vi "Authorize.vi"(6 "timeout (ms) [0: default]":i32, 8 "error in (no error)":errorcluster, 10 "State Parameter":string, 11 "Oauth2 in":refnum<class "Oauth2.lvclass">) -> (0 "error out":errorcluster, 2 "Access Token":string, 3 "Oauth2 out":refnum<class "Oauth2.lvclass">)   [LabVIEW 2017, in "Oauth2.lvclass"]
uses:
  Oauth2.lvclass
  OAuthToken/OAuth2 Token Element -- enum.ctl
  Oauth2.lvclass/Oauth2.ctl
  OAuth2 Grant Type -- ring.ctl
  <vilib>/LabVIEW Open Source Project/OpenURI/uri/URI.lvclass/URI.ctl
  OauthClient/OAuthClient.lvclass/OAuthClient.ctl
  <vilib>/LabVIEW Open Source Project/Connection/Connection.TCP/Connection.TCP.lvclass
  C:/Program Files (x86)/National Instruments/LabVIEW 2024/vi.lib/LabVIEW Open Source Project/Connection/Connection/Connection.lvclass
  <vilib>/LabVIEW Open Source Project/Connection/Connection/Connection.lvclass
  <vilib>/LabVIEW Open Source Project/OpenURI/uri/URI.lvclass
  OAuthToken/OAuthAccessToken.lvclass
  OauthClient/OAuthClient.lvclass
panel:
  in  "Status":string(combo)="400 BAD REQUEST"
  out "Request":string
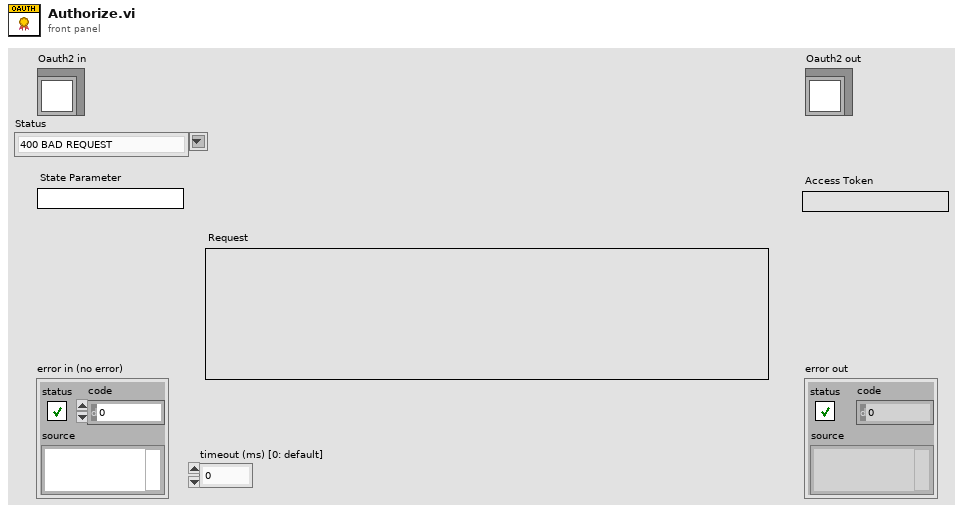
[diagram p1: front panel]
types:
  T1 = typedef "OAuthAccessToken.lvclass/OAuth2 Token Element -- enum.ctl" = enum16{"client_id", "client_secret", "response_type", "scope", "redirect_uri", "error", "error_description", "error_uri", "grant_type", "code", "access_token", "token_type", "expires_in", "username", "password", "refresh_token", "code_challenge", "code_challenge_method", "reverse_proxy_uri", "endpoint element", "access_type", "prompt", "id_token"}
  T2 = typedef "Oauth2.lvclass/OAuth2 Flow -- enum.ctl" = enum16{"Authorization Code", "Authorization Code (PKCE)", "Implicit", "Resource Owner Credentials", "Client Credentials"}
  T3 = typedef "Oauth2.lvclass/OAuth2 Grant Type -- ring.ctl" = string
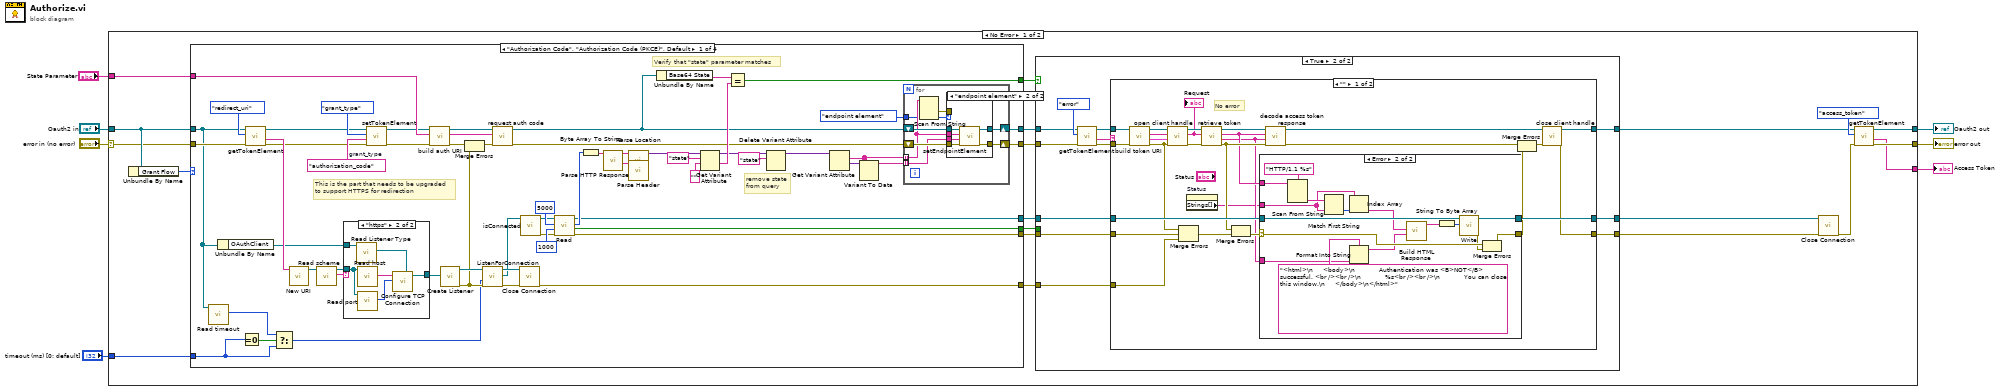
[diagram p0: block diagram]
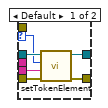
[diagram p2: hidden frame]
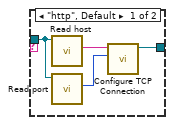
[diagram p3: hidden frame]
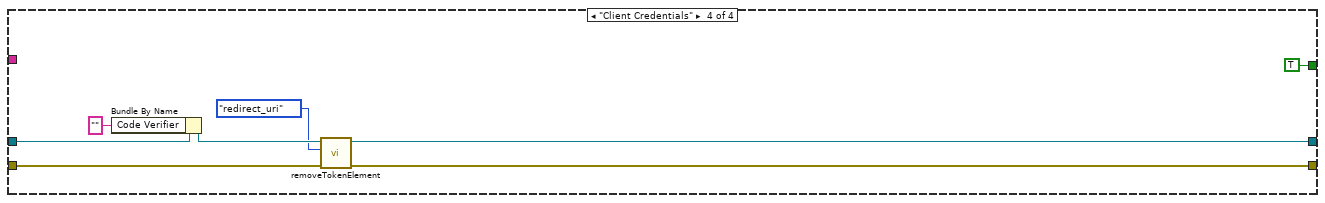
[diagram p6: hidden frame]
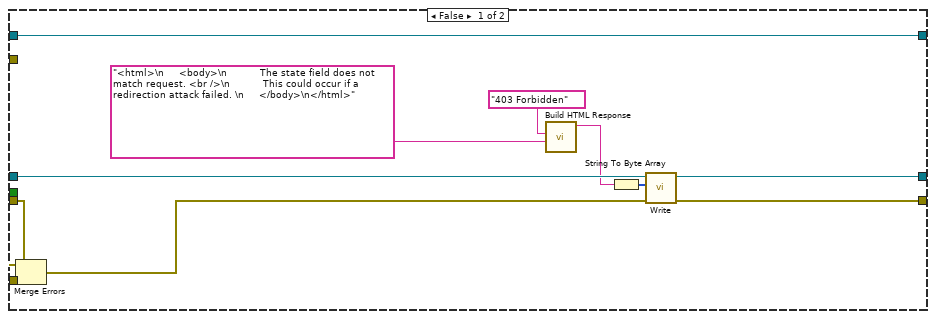
[diagram p7: hidden frame]
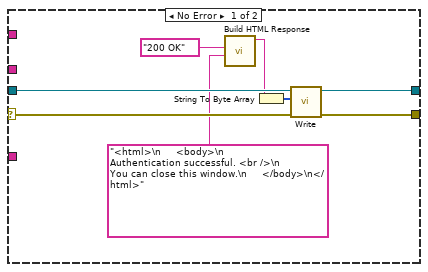
[diagram p8: hidden frame]
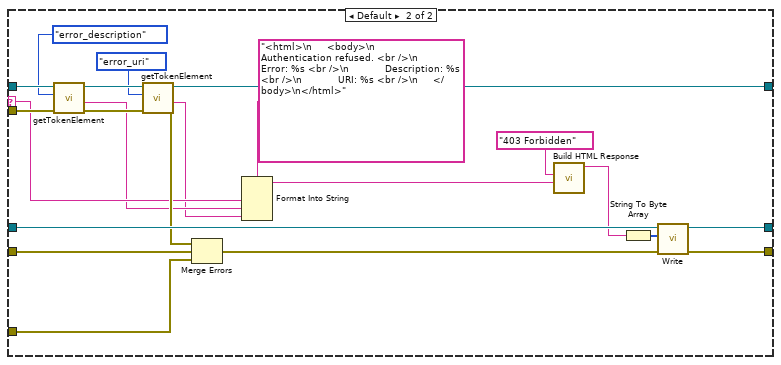
[diagram p9: hidden frame]
diagram:
  n1 = case shown="No Error" "error in (no error)" {
    selector: "error in (no error)" -> [w8 w226]
    tunnel: [w17 w226] -> w6
    tunnel: [w19 w225] -> w4
    tunnel: "Oauth2 in" -> [w9 w225]
    tunnel: "State Parameter" -> [w27 _]
    tunnel: [w14 _] -> w2
    tunnel: "timeout (ms) [0: default]" -> [w13 _]
    frame No Error {
      n2 = Unbundle By Name(w9) -> ("Grant Flow"=w10:T2)
      n3 = case shown="\"Authorization Code\", \"Authorization Code (PKCE)\", Default" w10 {
        tunnel: w27 -> [w83 _ _ _]
        tunnel: [w67 _ _ _] -> w25
        tunnel: [w66 _ _ _] -> w24
        tunnel: [w65 _ _ _] -> w23
        tunnel: [w61 _ _ TRUE] -> w21
        tunnel: [w60 _ _ _] -> w20
        tunnel: w13 -> [w43 _ _ _]
        tunnel: [w31 w118 w120 w122] -> w12
        tunnel: [w30 w117 w119 w121] -> w11
        tunnel: w8 -> [w29 w117 w119 w123]
        tunnel: w9 -> [w28 w118 w120 w127]
        frame "Authorization Code", "Authorization Code (PKCE)", Default {
          w46 = T3 "authorization_code"  # grant_type
          # "This is the part that needs to be upgraded\nto support HTTPS for redirection"
          # "remove state\nfrom query"
          # "Verify that \"state\" parameter matches"
          n4 = call "Read timeout.vi"("Oauth2 in"=w28) -> ("timeout (ms)"=w41:i32)  [unwired: 8 in, 2 out]
          n5 = Unbundle By Name(w28) -> ("OAuthClient"=w39:refnum<class "OAuthClient.lvclass">)
          n6 = Equal To 0?(x=w43) -> (x = 0?=w64:bool)
          n7 = call "getTokenElement.vi"("error in (no error)"=w29, "Token element"=OAuth2_Token_Element_--_enum."redirect_uri", "Oauth2 in"=w28) -> ("error out"=w42:errorcluster, "Value"=w58:string, "Oauth2 out"=w40:refnum<class "Oauth2.lvclass">)  [unwired: 4 in, 2 out]
          n8 = Select(t=w41, s=w64, f=w43) -> (s? t:f=w63:i32)
          n9 = call <vilib>:"New URI.vi"("URI"=w58) -> ("URI"=w57:refnum<class "URI.lvclass">)  [unwired: 9 in, 1 out]
          n10 = call <vilib>:"Read scheme.vi"("URI in"=w57) -> ("scheme"=w85:string, "URI out"=w84:refnum<class "URI.lvclass">)  [unwired: 8 in, 1 out]
          n11 = case shown="\"https\"" w85 {
            tunnel: w84 -> [w107 w113]
            tunnel: [w108 w114] -> w74
            tunnel: w39 -> [_ w112]
            frame "http", Default {
              n12 = call <vilib>:"Read host.vi"("URI in"=w107) -> ("host"=w110:string)  [unwired: 8 in, 2 out]
              n13 = call <vilib>:"Read port.vi"("URI in"=w107) -> ("port"=w109:u16)  [unwired: 8 in, 2 out]
              n14 = call <vilib>:"Configure TCP Connection.vi"("remote port (80)"=w109, "address (localhost)"=w110) -> ("Connection.TCP"=w108:refnum<class "Connection.TCP.lvclass">)  [unwired: 8 in, 1 out]
            }
            frame "https" {
              n15 = call "Read Listener Type.vi"("OAuthClient in"=w112) -> ("Listener Type"=w111:refnum<class "Connection.TCP.lvclass">)  [unwired: 8 in, 2 out]
              n16 = call <vilib>:"Read host.vi"("URI in"=w113) -> ("host"=w116:string)  [unwired: 8 in, 2 out]
              n17 = call <vilib>:"Read port.vi"("URI in"=w113) -> ("port"=w115:u16)  [unwired: 8 in, 2 out]
              n18 = call <vilib>:"Configure TCP Connection.vi"("Connection.TCP"=w111, "remote port (80)"=w115, "address (localhost)"=w116) -> ("Connection.TCP"=w114:refnum<class "Connection.TCP.lvclass">)  [unwired: 7 in, 1 out]
            }
          }
          n19 = call "setTokenElement.vi"("error in (no error)"=w42, "Value"=w46, "Token element"=OAuth2_Token_Element_--_enum."grant_type", "Oauth2 in"=w40) -> ("error out"=w44:errorcluster, "Oauth2 out"=w45:refnum<class "Oauth2.lvclass">)  [unwired: 6 in]
          n20 = call-dynamic "build auth URI.vi"("error in (no error)"=w44, "State Parameter"=w83, "Oauth2 in"=w45) -> ("error out"=w68:errorcluster, "Authorization Request URI"=w70:string, "Oauth2"=w69:refnum<class "Oauth2.lvclass">)  [unwired: 6 in]
          n21 = call <vilib>:"Create Listener.vi"("Connection Configuration"=w74) -> ("error out"=w72:errorcluster, "Listener"=w80:refnum<class "Connection.TCP.lvclass">)  [unwired: 9 in]
          n22 = Merge Errors(w68, w72) -> (w71:errorcluster)
          n23 = call <vilib>:"ListenForConnection.vi"("error in (no error)"=w72, "timeout (2000 ms)"=w63, "Listener"=w80) -> ("error out"=w82:errorcluster, "Connection"=w77:refnum<class "Connection.lvclass">, "Listener out"=w79:refnum<class "Connection.TCP.lvclass">)  [unwired: 5 in, 1 out]
          n24 = call-dynamic "request auth code.vi"("error in (no error)"=w71, "Request URI"=w70, "Oauth2 in"=w69) -> ("error out"=w33:errorcluster, "Oauth2 out"=w34:refnum<class "Oauth2.lvclass">)  [unwired: 7 in]
          n25 = call <vilib>:"Close Connection.vi"("error in (no error)"=w82, "Connection in"=w79) -> ("error out"=w66:errorcluster)  [unwired: 8 in, 1 out]
          n26 = call <vilib>:"isConnected.vi"("Connection in"=w77) -> ("error out"=w75:errorcluster, "Connection out"=w76:refnum<class "Connection.lvclass">)  [unwired: 8 in, 1 out]
          n27 = call <vilib>:"Read.vi"("error in (no error)"=w75, "timeout (2000 ms)"=1000 ("bytes to read (100)"), "bytes to read (100)"=5000, "TCPConnection in"=w76) -> ("error out"=w65:errorcluster, "timed out"=w60:bool, "Bytes"=w73:u8[], "TCPConnection out"=w67:refnum<class "Connection.lvclass">)  [unwired: 3 in, 1 out]
          n28 = Byte Array To String(unsigned byte array=w73) -> (string=w56:string)
          n29 = call "Parse HTTP Response.vi"("HTTP Response"=w56) -> ("Header"=w55:string, "Location"=w54:string)  [unwired: 5 in, 4 out]
          n30 = call "Parse Location.vi"("Location"=w54) -> ("Query Parameters"=w53:variant)  [unwired: 10 in]
          n31 = call "Parse Header.vi"("HTTP Header"=w55) -> ()  [unwired: 10 in, 1 out]
          n32 = Unbundle By Name(w34) -> ("Base64 State"=w62:string)
          n33 = Get Variant Attribute(Variant=w53, name="state", default value (empty Variant)="") -> (duplicate Variant=w49:variant, value=w50:string)  [unwired: 1 in, 2 out]
          n34 = Equal?(x=w62, y=w50) -> (x = y?=w61:bool)
          n35 = Delete Variant Attribute(6:"state", 7:w49) -> (3:w32:variant)  [unwired: 1 in, 2 out]
          n36 = Get Variant Attribute(Variant=w32) -> (names=w38:string[], values=w36:variant[])  [unwired: 3 in, 2 out]
          n37 = Variant To Data(type=w38, Variant=w36) -> (data=w37:string[])  [unwired: 1 in, 1 out]
          n38 = for {
            shift-right: [w92] -> w31
            shift-left: w34 -> [w93]
            shift-right: [w89] -> w30
            shift-left: w33 -> [w91]
            tunnel: w38 -> [w87] mode=indexing
            tunnel: w37 -> [w90] mode=indexing
            tunnel: OAuth2_Token_Element_--_enum."endpoint element" ("Token element") -> [w86]
            n39 = Scan From String(input string=w87, default 1=w86) -> (error out=w88:errorcluster, output 1=w94:T1)  [unwired: 3 in, 2 out]
            n40 = case shown="\"endpoint element\"" w94 {
              selector: w94 -> [w98 _]
              tunnel: w93 -> [w100 w106]
              tunnel: [w99 w105] -> w92
              tunnel: w91 -> [w97 w104]
              tunnel: w90 -> [w96 w102]
              tunnel: [w95 w103] -> w89
              tunnel: w88 -> [_ _]
              tunnel: w87 -> [_ w101]
              frame Default {
                n41 = call "setTokenElement.vi"("error in (no error)"=w97, "Value"=w96, "Token element"=w98, "Oauth2 in"=w100) -> ("error out"=w95:errorcluster, "Oauth2 out"=w99:refnum<class "Oauth2.lvclass">)  [unwired: 6 in]
              }
              frame "endpoint element" {
                n42 = call "setEndpointElement.vi"("error in (no error)"=w104, "Value"=w102, "Endpoint Name"=w101, "Oauth2 in"=w106) -> ("error out"=w103:errorcluster, "Oauth2 out"=w105:refnum<class "Oauth2.lvclass">)  [unwired: 6 in]
              }
            }
          }
        }
        frame "Implicit" {
        }
        frame "Resource Owner Credentials" {
        }
        frame "Client Credentials" {
          n43 = Bundle By Name(cluster=w127, "Code Verifier"="") -> (w126:refnum<class "Oauth2.lvclass">)
          n44 = call "removeTokenElement.vi"("error in (no error)"=w123, "Token element"=OAuth2_Token_Element_--_enum."redirect_uri", "Oauth2 in"=w126) -> ("error out"=w121:errorcluster, "Oauth2 out"=w122:refnum<class "Oauth2.lvclass">)  [unwired: 7 in]
        }
      }
      n45 = case shown="True" w21 {
        tunnel: w12 -> [w133 w142]
        tunnel: w11 -> [w132 w141]
        tunnel: [w138 w152] -> w26
        tunnel: w25 -> [w139 w151]
        tunnel: w24 -> [w136 w150]
        tunnel: w23 -> [w135 w149]
        tunnel: [w133 w148] -> w15
        tunnel: [w137 w147] -> w22
        tunnel: w20 -> [_ _]
        frame False {
          n46 = Merge Errors(w132, w135, w136) -> (w134:errorcluster)
          n47 = call "Build HTML Response.vi"("HTML"="<html>\n     <body>\n           The state field does not match request. <br />\n           This could occur if a redirection attack failed. \n     </body>\n</html>" ("regular expression"), "Status"="403 Forbidden") -> ("HTTP Response"=w129:string)  [unwired: 9 in]
          n48 = String To Byte Array(string=w129) -> (unsigned byte array=w140:u8[])
          n49 = call <vilib>:"Write.vi"("error in (no error)"=w134, "Bytes"=w140, "Connection in"=w139) -> ("error out"=w137:errorcluster, "Connection"=w138:refnum<class "Connection.lvclass">)  [unwired: 7 in]
        }
        frame True {
          n50 = call "getTokenElement.vi"("error in (no error)"=w141, "Token element"=OAuth2_Token_Element_--_enum."error", "Oauth2 in"=w142) -> ("error out"=w145:errorcluster, "Value"=w143:string, "Oauth2 out"=w146:refnum<class "Oauth2.lvclass">)  [unwired: 4 in, 2 out]
          n51 = case shown="\"\"" w143 {
            selector: w143 -> [_ w209]
            tunnel: [w178 w224] -> w152
            tunnel: w151 -> [w177 w222]
            tunnel: w150 -> [w176 w221]
            tunnel: w149 -> [w175 w220]
            tunnel: [w169 w214] -> w148
            tunnel: [w161 w219] -> w147
            tunnel: w146 -> [w160 w217]
            tunnel: w145 -> [w159 w212]
            frame "" {
              # "No error"
              n52 = call-dynamic "build token URI.vi"("error in (no error)"=w159, "Oauth2 in"=w160) -> ("error out"=w171:errorcluster, "Headers"=w158:cluster{"header":string, "value":string}[], "Token Request URI"=w172:string, "Oauth2"=w173:refnum<class "Oauth2.lvclass">)  [unwired: 6 in]
              n53 = call "open client handle.vi"("error in (no error)"=w171, "Headers"=w158, "Request URI in"=w172, "Oauth2 in"=w173) -> ("error out"=w167:errorcluster, "Request URI dup"=w166:string, "Oauth2 out"=w168:refnum<class "Oauth2.lvclass">)  [unwired: 5 in]
              "Request" <- w166
              n54 = Merge Errors(w171, w175, w176) -> (w174:errorcluster)
              n55 = property on="Status" class="CmbBox"() -> ("Strings[]"=w153:string[])  [unwired: 2 in, 2 out]
              n56 = call "retrieve token.vi"("error in (no error)"=w167, "Token Request URI"=w166, "Oauth2 in"=w168) -> ("error out"=w163:errorcluster, "Response"=w154:string, "Header"=w155:string, "Oauth2 out"=w165:refnum<class "Oauth2.lvclass">)  [unwired: 5 in]
              n57 = Merge Errors(w163, w174) -> (w156:errorcluster)
              n58 = case shown="Error" w156 {
                selector: w156 -> [w182 w199]
                tunnel: [w186 w202] -> w178
                tunnel: w177 -> [w184 w200]
                tunnel: [w183 w197] -> w157
                tunnel: w155 -> [_ w195]
                tunnel: w154 -> [_ w188]
                tunnel: w153 -> [_ w190]
                frame No Error {
                  n59 = call "Build HTML Response.vi"("HTML"="<html>\n     <body>\n            Authentication successful. <br />\n            You can close this window.\n     </body>\n</html>" ("regular expression"), "Status"="200 OK") -> ("HTTP Response"=w180:string)  [unwired: 9 in]
                  n60 = String To Byte Array(string=w180) -> (unsigned byte array=w185:u8[])
                  n61 = call <vilib>:"Write.vi"("error in (no error)"=w182, "Bytes"=w185, "Connection in"=w184) -> ("error out"=w183:errorcluster, "Connection"=w186:refnum<class "Connection.lvclass">)  [unwired: 7 in]
                }
                frame Error {
                  n62 = Scan From String(format string="HTTP/1.1 %s", input string=w195) -> (output 1=w193:string)  [unwired: 3 in, 3 out]
                  n63 = Match First String(2:w190, 3:w193) -> (0:w192:i32)  [unwired: 1 out]
                  n64 = Index Array(array=w190, index=w192) -> (element=w191:string)
                  n65 = Format Into String(format string="<html>\n     <body>\n            Authentication was <B>NOT</B> successful. <br /><br />\n            %s<br /><br />\n            You can close this window.\n     </body>\n</html>" ("regular expression"), w188) -> (resulting string=w187:string)  [unwired: 2 in, 1 out]
                  n66 = call "Build HTML Response.vi"("HTML"=w187, "Status"=w191) -> ("HTTP Response"=w196:string)  [unwired: 9 in]
                  n67 = String To Byte Array(string=w196) -> (unsigned byte array=w201:u8[])
                  n68 = call <vilib>:"Write.vi"("Bytes"=w201, "Connection in"=w200) -> ("error out"=w198:errorcluster, "Connection"=w202:refnum<class "Connection.lvclass">)  [unwired: 8 in]
                  n69 = Merge Errors(w199, w198) -> (w197:errorcluster)
                }
              }
              n70 = call-dynamic "decode access token response.vi"("error in (no error)"=w163, "Response"=w154, "Header"=w155, "Oauth2 in"=w165) -> ("error out"=w162:errorcluster, "Oauth2"=w164:refnum<class "Oauth2.lvclass">)  [unwired: 6 in]
              n71 = Merge Errors(w162, w157) -> (w170:errorcluster)
              n72 = call "close client handle.vi"("error in (no error)"=w170, "Oauth2 in"=w164) -> ("error out"=w161:errorcluster, "Oauth2 out"=w169:refnum<class "Oauth2.lvclass">)  [unwired: 8 in]
            }
            frame Default {
              n73 = call "getTokenElement.vi"("error in (no error)"=w212, "Token element"=OAuth2_Token_Element_--_enum."error_description", "Oauth2 in"=w217) -> ("error out"=w213:errorcluster, "Value"=w208:string, "Oauth2 out"=w215:refnum<class "Oauth2.lvclass">)  [unwired: 4 in, 2 out]
              n74 = call "getTokenElement.vi"("error in (no error)"=w213, "Token element"=OAuth2_Token_Element_--_enum."error_uri", "Oauth2 in"=w215) -> ("error out"=w211:errorcluster, "Value"=w207:string, "Oauth2 out"=w214:refnum<class "Oauth2.lvclass">)  [unwired: 4 in, 2 out]
              n75 = Merge Errors(w211, w220, w221) -> (w218:errorcluster)
              n76 = Format Into String(format string="<html>\n     <body>\n            Authentication refused. <br />\n            Error: %s <br />\n            Description: %s <br />\n            URI: %s <br />\n     </body>\n</html>" ("regular expression"), w209, w208, w207) -> (resulting string=w204:string)  [unwired: 2 in, 1 out]
              n77 = call "Build HTML Response.vi"("HTML"=w204, "Status"="403 Forbidden") -> ("HTTP Response"=w203:string)  [unwired: 9 in]
              n78 = String To Byte Array(string=w203) -> (unsigned byte array=w223:u8[])
              n79 = call <vilib>:"Write.vi"("error in (no error)"=w218, "Bytes"=w223, "Connection in"=w222) -> ("error out"=w219:errorcluster, "Connection"=w224:refnum<class "Connection.lvclass">)  [unwired: 7 in]
            }
          }
        }
      }
      n80 = call <vilib>:"Close Connection.vi"("error in (no error)"=w22, "Connection in"=w26) -> ("error out"=w18:errorcluster)  [unwired: 8 in, 1 out]
      n81 = call "getTokenElement.vi"("error in (no error)"=w18, "Token element"=OAuth2_Token_Element_--_enum."access_token", "Oauth2 in"=w15) -> ("error out"=w17:errorcluster, "Value"=w14:string, "Oauth2 out"=w19:refnum<class "Oauth2.lvclass">)  [unwired: 4 in, 2 out]
    }
    frame Error {
    }
  }
  "error out" <- w6
  "Oauth2 out" <- w4
  "Access Token" <- w2
